vi "VFF.vi"(7 "Max object avoidance distance":dbl, 8 "Target Angle":dbl, 9 "Target Magnitude":dbl, 10 "Object Magnitudes":dbl[](array[numeric]), 11 "Object Angles":dbl[](array[numeric])) -> (3 "Direction to move in":dbl)   [LabVIEW 2016]
panel:
  out "Force to move away from":dbl
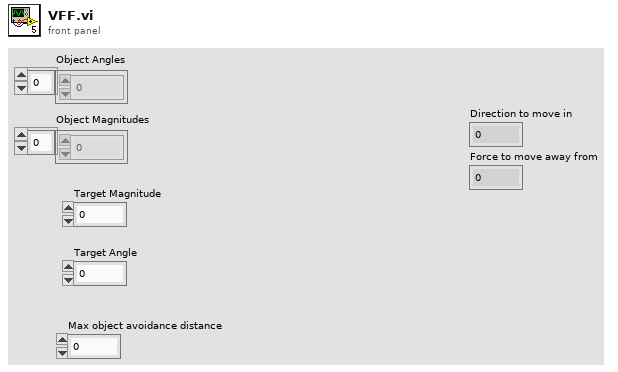
[diagram p1: front panel]
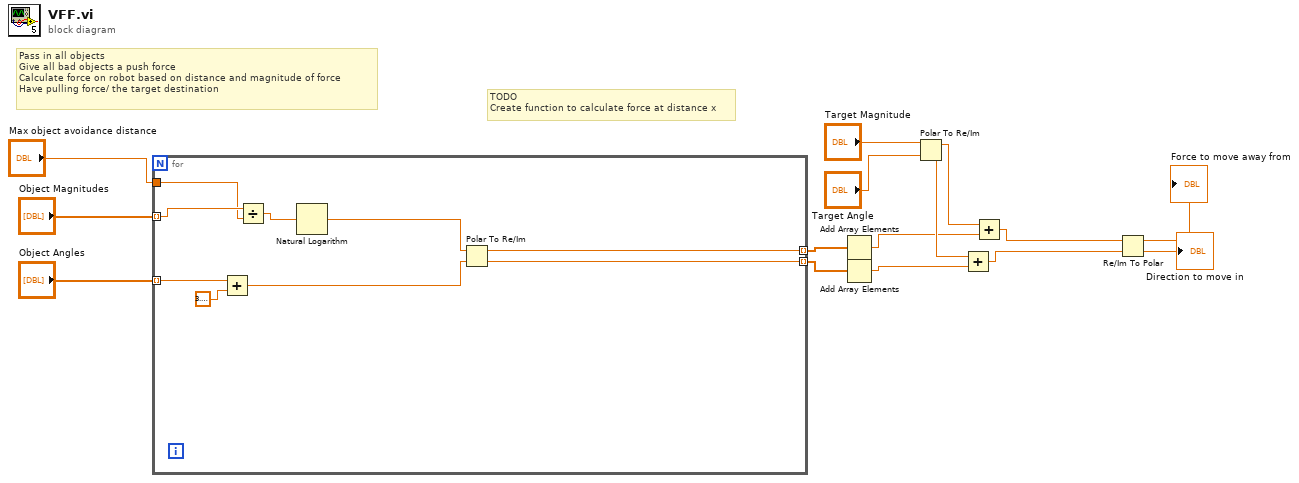
[diagram p0: block diagram]
diagram:
  # "TODO \nCreate function to calculate force at distance x"
  # "Pass in all objects\nGive all bad objects a push force\nCalculate force on robot based on distance and magnitude of force \nHave pulling force/ the target destination"
  n1 = for {
    tunnel: "Object Magnitudes" -> [w22] mode=indexing
    tunnel: "Object Angles" -> [w24] mode=indexing
    tunnel: "Max object avoidance distance" -> [w21]
    tunnel: [w17] -> w12 mode=indexing
    tunnel: [w16] -> w11 mode=indexing
    n2 = Add(x=w24, y=3.141592653589793) -> (x+y=w18:dbl)
    n3 = Divide(x=w22, y=w21) -> (x/y=w20:dbl)
    n4 = Natural Logarithm(1:w20) -> (0:w19:dbl)
    n5 = Polar To Re/Im(2:w18, 3:w19) -> (0:w16:dbl, 1:w17:dbl)
  }
  n6 = Add Array Elements(numeric array=w12) -> (sum=w6:dbl)
  n7 = Add Array Elements(numeric array=w11) -> (sum=w5:dbl)
  n8 = Polar To Re/Im(2:"Target Angle", 3:"Target Magnitude") -> (0:w7:dbl, 1:w8:dbl)
  n9 = Add(x=w7, y=w5) -> (x+y=w3:dbl)
  n10 = Add(x=w8, y=w6) -> (x+y=w4:dbl)
  n11 = Re/Im To Polar(2:w3, 3:w4) -> (0:→"Direction to move in":dbl, 1:→"Force to move away from":dbl)
